vi "Write Inclinometer Obj.vi"(8 "error in (no error)":errorcluster, 10 "Hardware.lvlib:Inclinometer.lvlib:Inclinometer.lvclass":refnum<class "Inclinometer.lvclass">, 11 "Inclinometer Configuration in":refnum<class "Inclinometer Configuration.lvclass">) -> (0 "error out":errorcluster, 3 "Inclinometer Configuration out":refnum<class "Inclinometer Configuration.lvclass">)   [LabVIEW 2016, in "Hardware.lvlib" / "Inclinometer.lvlib" / "Inclinometer Configuration.lvclass"]
uses:
  <userlib>/Common Components/Hardware/Inclinometer/Inclinometer Config/Inclinometer Configuration.lvclass
  <userlib>/Common Components/Hardware/Inclinometer/Inclinometer/Inclinometer.lvclass
  <userlib>/Common Components/Hardware/Inclinometer/Inclinometer Config/Inclinometer Configuration.lvclass/Inclinometer Configuration.ctl
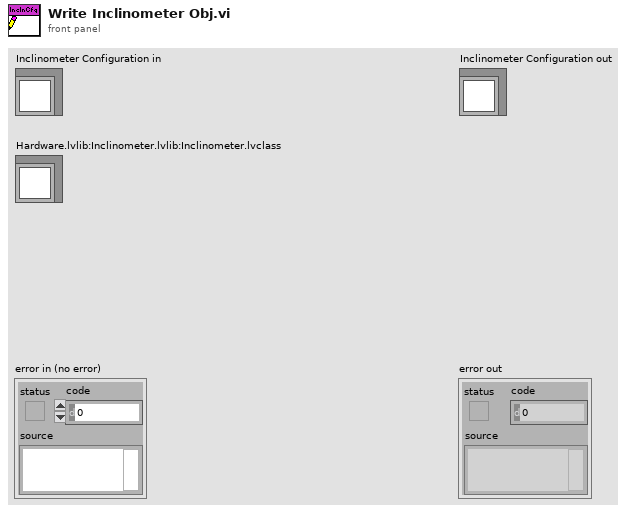
[diagram p1: front panel]
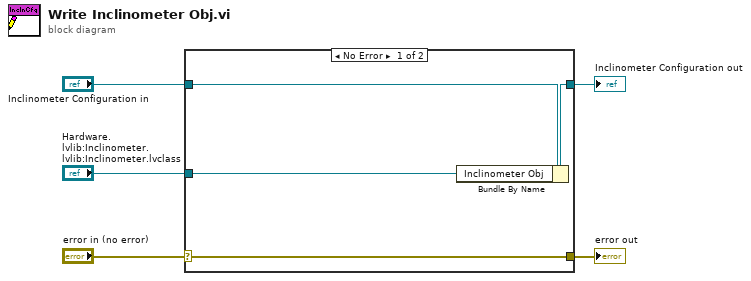
[diagram p0: block diagram]
diagram:
  n1 = case shown="No Error" "error in (no error)" {
    selector: "error in (no error)" -> [w9 w10]
    tunnel: [w9 w10] -> w4
    tunnel: [w7 w11] -> w2
    tunnel: "Inclinometer Configuration in" -> [w8 w11]
    tunnel: "Hardware.lvlib:Inclinometer.lvlib:Inclinometer.lvclass" -> [w6 _]
    frame No Error {
      n2 = Bundle By Name(cluster=w8, "Inclinometer Obj"=w6) -> (w7:refnum<class "Inclinometer Configuration.lvclass">)
    }
    frame Error {
    }
  }
  "error out" <- w4
  "Inclinometer Configuration out" <- w2
